vi "Configure Digital Output Signal.vi"(5 "Signal Type (0: I/Q)":i32(ring) items=["I/Q", "IF"], 6 "Scaling (70 %)":dbl=70.0, 7 "Rotation (0 deg)":dbl, 8 "error in (no error)":errorcluster, 9 "Q Offset (0 %)":dbl, 10 "I Offset (0 %)":dbl, 11 "VISA resource name":refnum<visa-resource-name>) -> (0 "error out":errorcluster, 3 "VISA resource name out":refnum<visa-resource-name>)   [LabVIEW 2018, in "Agilent PSG MXG Series.lvlib"]
doc: "Configures the N5102A module output mode.\n\n<b>Note:</b>\n(1) It is applicable for N5172B/82B with <b>Option 003<b> or <b>Option 004</b> or <b>both</b> only.\n(2) It is valid only for the N5102A output."
uses:
  Agilent PSG MXG Series.lvlib
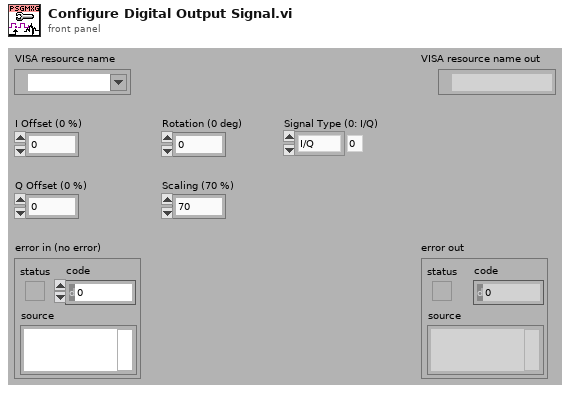
[diagram p1: front panel]
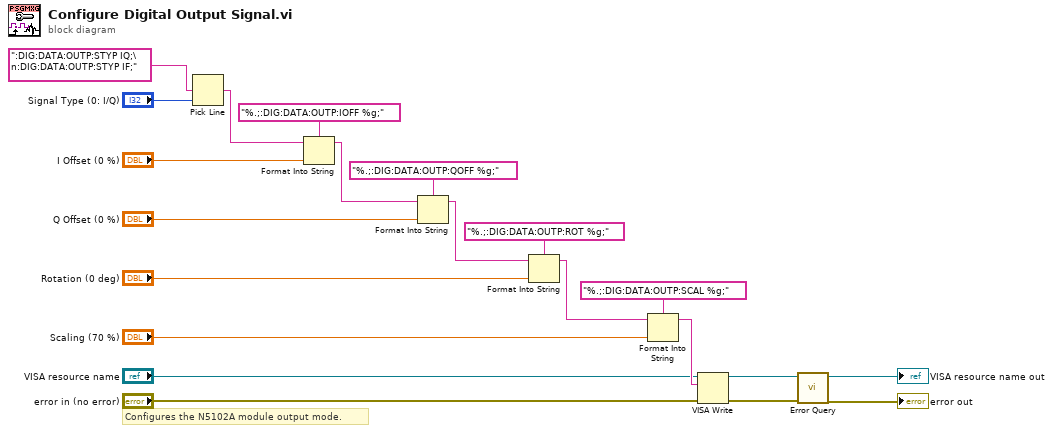
[diagram p0: block diagram]
diagram:
  # "Configures the N5102A module output mode."
  n1 = Pick Line(multi-line string=":DIG:DATA:OUTP:STYP IQ;\n:DIG:DATA:OUTP:STYP IF;", line index="Signal Type (0: I/Q)") -> (output string=w19:string)  [unwired: 1 in]
  n2 = Format Into String(format string="%.;:DIG:DATA:OUTP:IOFF %g;", initial string=w19, "I Offset (0 %)") -> (resulting string=w16:string)  [unwired: 1 in, 1 out]
  n3 = Format Into String(format string="%.;:DIG:DATA:OUTP:QOFF %g;", initial string=w16, "Q Offset (0 %)") -> (resulting string=w13:string)  [unwired: 1 in, 1 out]
  n4 = Format Into String(format string="%.;:DIG:DATA:OUTP:ROT %g;", initial string=w13, "Rotation (0 deg)") -> (resulting string=w10:string)  [unwired: 1 in, 1 out]
  n5 = Format Into String(format string="%.;:DIG:DATA:OUTP:SCAL %g;", initial string=w10, "Scaling (70 %)") -> (resulting string=w7:string)  [unwired: 1 in, 1 out]
  n6 = VISA Write(VISA resource name="VISA resource name", write buffer=w7, error in (no error)="error in (no error)") -> (VISA resource name out=w4:refnum<visa-resource-name>, error out=w3:errorcluster)  [unwired: 1 out]
  n7 = call "Error Query.vi"("error in (no error)"=w3, "VISA resource name"=w4) -> ("error out"=→"error out":errorcluster, "VISA resource name out"=→"VISA resource name out":refnum<visa-resource-name>)  [unwired: 6 in, 2 out]
